vi "Get Search Result.vi"(8 "error in (no error)":errorcluster, 11 "Composite Object in":refnum<class "CConfig Object.lvclass">) -> (0 "error out":errorcluster, 1 "deleted portion":i32, 2 "empty?":bool, 3 "Composite Object out":refnum<class "CConfig Object.lvclass">)   [LabVIEW 2013, in "CConfig Object.lvclass"]
doc: "Copyright 2018, Carya Automatisering, Wiebe Walstra."
uses:
  CConfig Object.lvclass
  CConfig Object.lvclass/CConfig Object.ctl
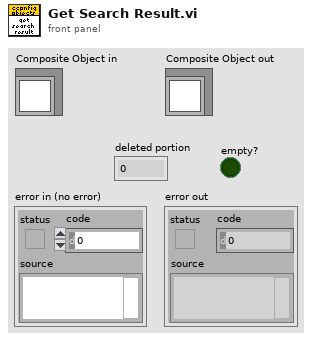
[diagram p1: front panel]
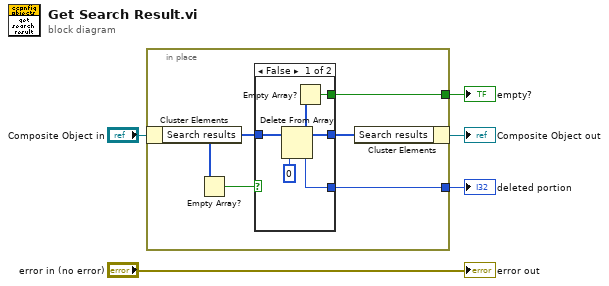
[diagram p0: block diagram]
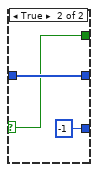
[diagram p2: hidden frame]
diagram:
  n1 = in-place {
    in-place-border: [w10] -> w4
    in-place-border: [w6] -> w1
    n2 = in-place-cluster #1("Composite Object in") -> ("Search results"=w9:i32[])
    n3 = Empty Array?(array=w9) -> (empty?=w8:bool)
    n4 = case shown="False" w8 {
      selector: w8 -> [_ w16]
      tunnel: [w14 -1 ("Numeric")] -> w10
      tunnel: w9 -> [w13 w18]
      tunnel: [w12 w18] -> w7
      tunnel: [w11 w16] -> w6
      frame False {
        n5 = Delete From Array(array=w13, index=0) -> (deleted portion=w14:i32, array with subset deleted=w12:i32[])  [unwired: 1 in]
        n6 = Empty Array?(array=w12) -> (empty?=w11:bool)
      }
      frame True {
      }
    }
    n7 = in-place-cluster #1("Search results"=w7) -> (→"Composite Object out":refnum<class "CConfig Object.lvclass">)
  }
  "deleted portion" <- w4
  "empty?" <- w1
  "error out" <- "error in (no error)"
